vi "Autonomous Independent.vi"   [LabVIEW 2014]
doc: "This VI is called when autonomous begins, and will automatically be terminated when autonomous ends. You can carry out timed or sensor driven robot movement independently without needing to return to the caller."
uses:
  <vilib>/Rock Robotics/Network Tables/SD Write Number.vi
  <vilib>/Rock Robotics/WPI/RobotDrive/WPI_RobotDriveGetSetRefNum.vi
  <vilib>/Rock Robotics/WPI/RobotDrive/WPI_RobotDriveArcadeDrive_Standard(NoSaturation).vi
  <vilib>/Rock Robotics/Network Tables/SD Write Numeric Array.vi
  <vilib>/Rock Robotics/Network Tables/SD Write Boolean.vi
panel:
  # "Be sure to right-click and choose Data Operations>>Make Current Value default if you want to save the array values with the VI"
types:
  T1 = typedef "WPI_MotorControlDeviceRef.ctl" = cluster{"DeviceStatus":errorcluster, "Type":T2, "PWM":cluster{"Controller":T3, "PWM Channel":T4, "DeadBand":T5}, "CAN":cluster{"Device Number":u8, "Control Mode":T6, "Semaphore":T7, "Max Vout":dbl, "TalonSRX Control Mode":T8}, "Invert":bool, "TransformRef":T9, "InvTransformRef":T9}
  T2 = typedef "WPI_MotorControlType.ctl" = enum16{"PWM", "CAN", "CANTalonSRX"}
  T3 = typedef "FPGA_TypedefDigitalModule.ctl" = enum16{"Controller 1"}
  T4 = typedef "FPGA_DIOPWMChannel.ctl" = enum8{"PWM 0", "PWM 1", "PWM 2", "PWM 3", "PWM 4", "PWM 5", "PWM 6", "PWM 7", "PWM 8", "PWM 9", "PWM MXP 0", "PWM MXP 1", "PWM MXP 2", "PWM MXP 3", "PWM MXP 4", "PWM MXP 5", "PWM MXP 6", "PWM MXP 7", "PWM MXP 8", "PWM MXP 9", "Invalid"}
  T5 = typedef "WPI_PWMDeadband.ctl" = cluster{"Name":string, "maxPositivePwm":i32, "minPositivePwm":i32, "centerPwm":i32, "maxNegativePwm":i32, "minNegativePwm":i32, "angularRange":u16}
  T6 = typedef "WPI_CANJaguar_ControlMode.ctl" = enum8{"Percent VBus", "Current", "Speed", "Position", "Voltage"}
  T7 = typedef "Semaphore RefNum" = refnum<k1>
  T8 = typedef "WPI_CANTalonSRX_APIControlMode.ctl" = enum8{"Percent VBus", "Speed", "Position", "Slave", "Unchanged / Invalid"}
  T9 = typedef "WPI_PWMTransform_ConPane.ctl" = refnum<vi>
  T10 = typedef "WPI_EncoderDevRef.ctl" = cluster{"DevStatus":errorcluster, "EncoderIndex":T11, "CounterIndex":T12, "DistancePerCount":dbl, "Decoding Type":T13}
  T11 = typedef "FPGA_EncoderIdx.ctl" = enum8{"Enc 0", "Enc 1", "Enc 2", "Enc 3", "Enc 4", "Enc 5", "Enc 6", "Enc 7", "Invalid"}
  T12 = typedef "FPGA_CounterCtrSystemIndex.ctl" = enum8{"Ctr 0", "Ctr 1", "Ctr 2", "Ctr 3", "Ctr 4", "Ctr 5", "Ctr 6", "Ctr 7", "Invalid"}
  T13 = typedef "WPI_EncoderType.ctl" = enum16{"1x", "2x", "4x"}
  T14 = typedef "WPI_RobotDriveDevRef.ctl" = cluster{"DevStatus":errorcluster, "Motors[]":T1[], "Square Inputs":bool, "Max Output":dbl}
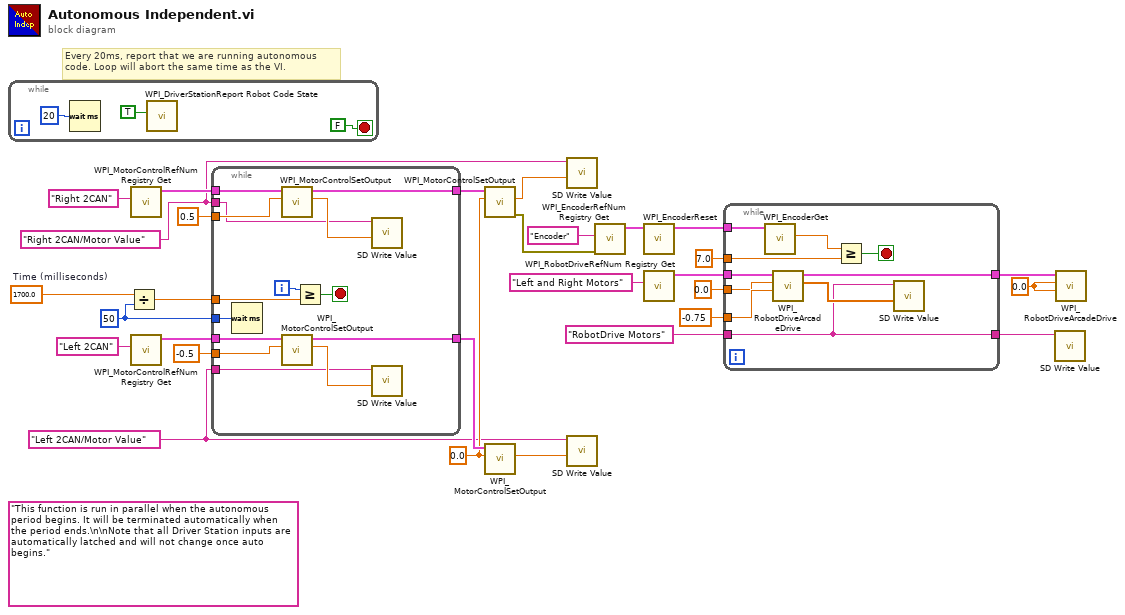
[diagram p0: block diagram]
diagram:
  w4 = 0.0 ("X axis value")
  w14 = "Left 2CAN/Motor Value" ("Name")
  w15 = "Right 2CAN/Motor Value" ("Name")
  w18 = 0.0 ("Output")
  w21 = 50
  w23 = 1700.0  # Time (milliseconds)
  (unwired) "This function is run in parallel when the autonomous period begins. It will be terminated automatically when the period ends.\n\nNote that all Driver Station inputs are automatically latched and will not change once auto begins."
  # "Every 20ms, report that we are running autonomous\ncode. Loop will abort the same time as the VI."
  n1 = while {
    stop <- FALSE stop-if-true
    n2 = Wait (ms)(milliseconds to wait=u32 20) -> ()  [unwired: 1 out]
    n3 = call <vilib>:"WPI_DriverStationReport Robot Code State.vi"("Autonomous"=TRUE) -> ()  [unwired: 10 in, 1 out]
  }
  n4 = Divide(x=w23, y=w21) -> (x/y=w22:dbl)
  n5 = call <vilib>:"WPI_MotorControlRefNum Registry Get.vi"("refnum name"="Right 2CAN") -> ("MotorControlDevRef"=w24:T1)  [unwired: 9 in, 1 out]
  n6 = call <vilib>:"WPI_MotorControlRefNum Registry Get.vi"("refnum name"="Left 2CAN") -> ("MotorControlDevRef"=w27:T1)  [unwired: 9 in, 1 out]
  n7 = while {
    tunnel: w22 -> [w45]
    tunnel: w27 -> [w43]
    tunnel: -0.5 ("Output") -> [w42]
    tunnel: 0.5 ("Output") -> [w41]
    tunnel: w24 -> [w40]
    tunnel: w21 -> [w39]
    tunnel: [w38] -> w20
    tunnel: [w37] -> w19
    tunnel: w15 -> [w34]
    tunnel: w14 -> [w33]
    i -> [w44]
    stop <- w46 stop-if-true
    n8 = Wait (ms)(milliseconds to wait=w39) -> ()  [unwired: 1 out]
    n9 = call <vilib>:"WPI_MotorControlSetOutput.vi"("Output"=w41, "MotorControlDevRef"=w40) -> ("Motor Output"=w36:dbl, "MotorControlDevRef"=w38:T1)  [unwired: 7 in, 1 out]
    n10 = call <vilib>:"WPI_MotorControlSetOutput.vi"("Output"=w42, "MotorControlDevRef"=w43) -> ("Motor Output"=w35:dbl, "MotorControlDevRef"=w37:T1)  [unwired: 7 in, 1 out]
    n11 = Greater Or Equal?(x=w44, y=w45) -> (x >= y?=w46:bool)
    n12 = call-poly <vilib>:"SD Write Value.vi"("Numeric"=w36, "Name"=w34) -> ()  [unwired: 8 in, 2 out]
    n13 = call-poly <vilib>:"SD Write Value.vi"("Numeric"=w35, "Name"=w33) -> ()  [unwired: 8 in, 2 out]
  }
  n14 = call <vilib>:"WPI_MotorControlSetOutput.vi"("Output"=w18, "MotorControlDevRef"=w20) -> ("error out"=w7:errorcluster, "Motor Output"=w17:dbl)  [unwired: 7 in, 1 out]
  n15 = call <vilib>:"WPI_MotorControlSetOutput.vi"("Output"=w18, "MotorControlDevRef"=w19) -> ("Motor Output"=w16:dbl)  [unwired: 7 in, 2 out]
  n16 = call-poly <vilib>:"SD Write Value.vi"("Numeric"=w17, "Name"=w15) -> ()  [unwired: 8 in, 2 out]
  n17 = call-poly <vilib>:"SD Write Value.vi"("Numeric"=w16, "Name"=w14) -> ()  [unwired: 8 in, 2 out]
  n18 = call <vilib>:"WPI_EncoderRefNum Registry Get.vi"("error in (no error)"=w7, "refnum name"="Encoder") -> ("EncoderDevRef"=w13:T10)  [unwired: 8 in, 1 out]
  n19 = call <vilib>:"WPI_EncoderReset.vi"("EncoderDevRef"=w13) -> ("EncoderDevRef"=w11:T10)  [unwired: 9 in, 1 out]
  n20 = call <vilib>:"WPI_RobotDriveRefNum Registry Get.vi"("refnum name"="Left and Right Motors") -> ("RobotDriveDevRef"=w8:T14)  [unwired: 1 in, 9 out]
  n21 = while {
    tunnel: w11 -> [w55]
    tunnel: "RobotDrive Motors" ("Name") -> [w50]
    tunnel: w8 -> [w52]
    tunnel: 7.0 ("Numeric") -> [w51]
    tunnel: [w50] -> w6
    tunnel: [w49] -> w5
    tunnel: -0.75 ("Y axis value") -> [w48]
    tunnel: 0.0 ("X axis value") -> [w47]
    stop <- w56 stop-if-true
    n22 = call <vilib>:"WPI_EncoderGet.vi"("EncoderDevRef"=w55) -> ("Distance"=w53:dbl)  [unwired: 5 in, 5 out]
    n23 = call-poly <vilib>:"WPI_RobotDriveArcadeDrive.vi"("Y axis value"=w48, "X axis value"=w47, "RobotDriveDevRef"=w52) -> ("Motor Values"=w54:dbl[], "RobotDriveDevRef"=w49:T14)  [unwired: 6 in, 1 out]
    n24 = Greater Or Equal?(x=w53, y=w51) -> (x >= y?=w56:bool)
    n25 = call-poly <vilib>:"SD Write Value.vi"("Numeric Array"=w54, "Name"=w50) -> ()  [unwired: 8 in, 2 out]
  }
  n26 = call-poly <vilib>:"SD Write Value.vi"("Name"=w6) -> ()  [unwired: 9 in, 2 out]
  n27 = call-poly <vilib>:"WPI_RobotDriveArcadeDrive.vi"("Y axis value"=w4, "X axis value"=w4, "RobotDriveDevRef"=w5) -> ()  [unwired: 6 in, 3 out]
